vi "example_06_data_entry_numeric.vi"() -> ()   [LabVIEW 2015, in "lv-dialog.lvlib" / "v1.lvlib"]
uses:
  v1.lvlib
  public/_controls/selection.ctl
  public/class/v1.lvclass
panel:
  in  "boolean_text_2":string="Cancel"
  out "data":dbl
  in  "boolean_text_1":string="OK"
  in  "dialog_text":string="Enter a number"
  out "error":errorcluster
  out "dialog_selection":T1
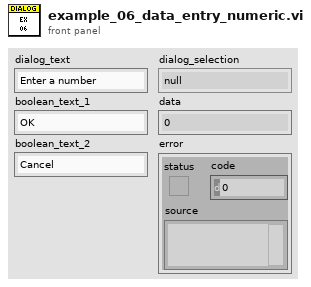
[diagram p1: front panel]
types:
  T1 = typedef "lv-dialog.lvlib/v1.lvlib/selection.ctl" = enum16{"null", "panel_closed", "button_1", "button_2", "button_3", "cancelled"}
  T2 = cluster{"dialog_text":string, "boolean_text_1":string, "boolean_text_2":string}
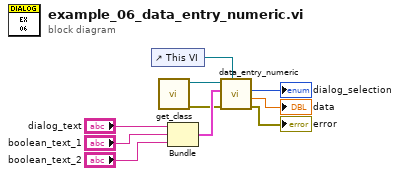
[diagram p0: block diagram]
diagram:
  n1 = control-ref of="This VI"() -> (w4:refnum<vi>)
  n2 = call "get_class.vi"() -> ("error out"=w6:errorcluster, "class"=w7:refnum<class "v1.lvclass">)  [unwired: 10 in]
  n3 = Bundle("dialog_text"="dialog_text", "boolean_text_1"="boolean_text_1", "boolean_text_2"="boolean_text_2") -> (w8:T2)  [unwired: 1 in]
  n4 = call-dynamic "data_entry_numeric.vi"("callee"=w4, "error in (no error)"=w6, "configuration"=w8, "v1 in"=w7) -> ("error out"=→"error":errorcluster, "data"=→"data":dbl, "dialog_selection"=→"dialog_selection":T1)  [unwired: 4 in, 1 out]
